vi "ShamStimSimple.vi"(0 "event in port":u16=5557, 5 "event in channel":u16=1 min=1 max=8, 7 "Digital sham stim channel":tag="PCI-DAQ/port0/line0") -> (4 "New event":bool, 6 "Time on (samp.)":i64, 8 "Crossing time":i64, 10 "Crossing level":sgl, 13 "Phase threshold":sgl(graph)=145.96965, 14 "Learning rate (for adaptive threshold)":dbl(graph)=0.005000000792214087)   [LabVIEW 2017]
uses:
  <vilib>/Platform/TimedLoop/XDataNode/timing_clust.ctl
  <vilib>/Platform/TimedLoop/XDataNode/nitl_modes.ctl
  <vilib>/Platform/TimedLoop/XDataNode/wakeup.ctl
  <vilib>/DAQmx/write.llb/DAQmx Write (Digital Bool 1Line 1Point).vi
  <vilib>/DAQmx/miscellaneous.llb/DAQmx Fill In Error Info.vi
  <vilib>/platform/TimedLoop/XDataNode/XDataNode.xnode
  <vilib>/addons/zeromq/zmq_socket.lvclass
  <vilib>/Platform/TimedLoop/XDataNode/XDNodeRunTimeDep.lvlib
panel:
  out "last run error":errorcluster
  in  "event out channel":u16=3
  in  "Output type":enum16{"DAQ Digital Out", "Network Event"}(ring)=enum."Network Event"
  in  "event out port":u16=5556
  in  "stop":bool
  in  "Run":bool
  # "*** Start OpenEphys acquisition before the VI. ***"
  # "*** In the audio settings in the OpenEphys GUI, reduce the buffer size to get a 10 ms buffer period.  If ASIO is installed and enabled in\nthe Open Ephys build, use ASIO with sample rate (in audio settings) = 192,000 Hz and buffer size = 192 (1 ms buffer period). ***"
  # "Settings only take effect\nnext time a run is started."
  # "If output type is \"Network Event\":"
  # "If output type is \"DAQ Digital Out\":"
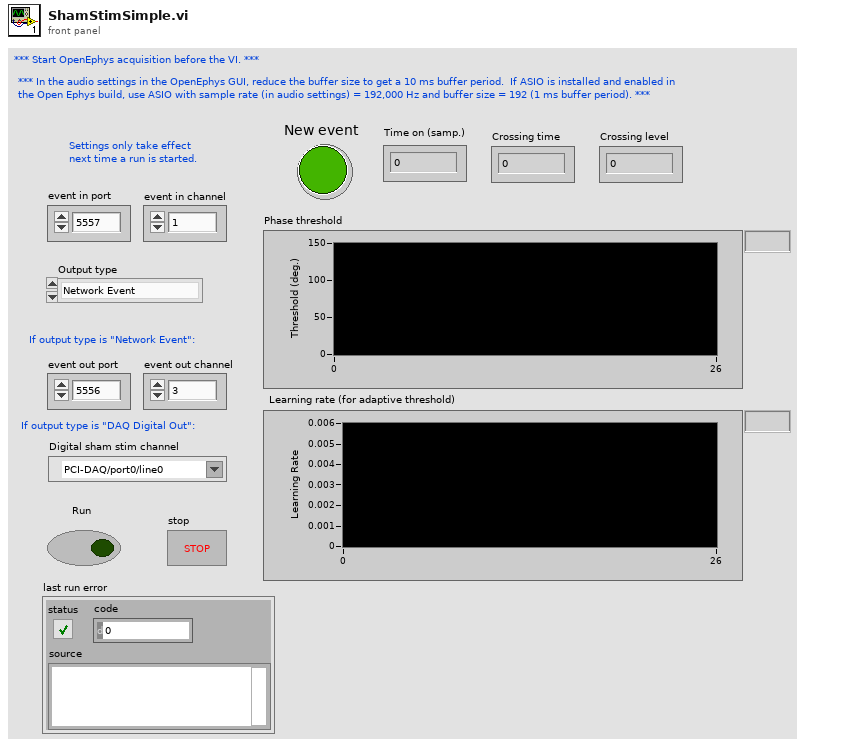
[diagram p1: front panel]
types:
  T1 = typedef "XDNodeRunTimeDep.lvlib/timing_clust.ctl" = cluster{"Expected End [f-1]":u64, "Actual End [f-1]":u64, "Finished Late? [f-1]":bool, "Expected End [i-1]":u64, "Actual End [i-1]":u64, "Finished Late? [i-1]":bool, "Expected Start [i]":u64, "Actual Start [i]":u64, "Expected Start [f]":u64, "Actual Start [f]":u64, "Source Name":string, "Structure Name":string, "Period":i64, "Deadline":i64, "Offset":i64, "Start":i64, "Priority":i32, "Timeout":i32, "Mode":T2, "Wakeup Reason":T3, "Error":errorcluster, "Source Type":string, "Secondary Source Type":string, "Global End Time":u64, "Global Start Time":u64, "Frame Duration":u64, "Iteration Duration":u64, "Assigned CPU":i32, "I/O Scan Engine Mode":u32}
  T2 = typedef "XDNodeRunTimeDep.lvlib/nitl_modes.ctl" = enum32{"No Change", "Process missed periods, maintain original phase", "Discard missed periods, maintain original phase", "Process missed periods, ignore original phase", "Discard missed periods, ignore original phase"}
  T3 = typedef "XDNodeRunTimeDep.lvlib/wakeup.ctl" = enum32{"Normal", "Aborted", "Asynchronous wakeup", "Timing source error", "Timed loop error", "Timeout"}
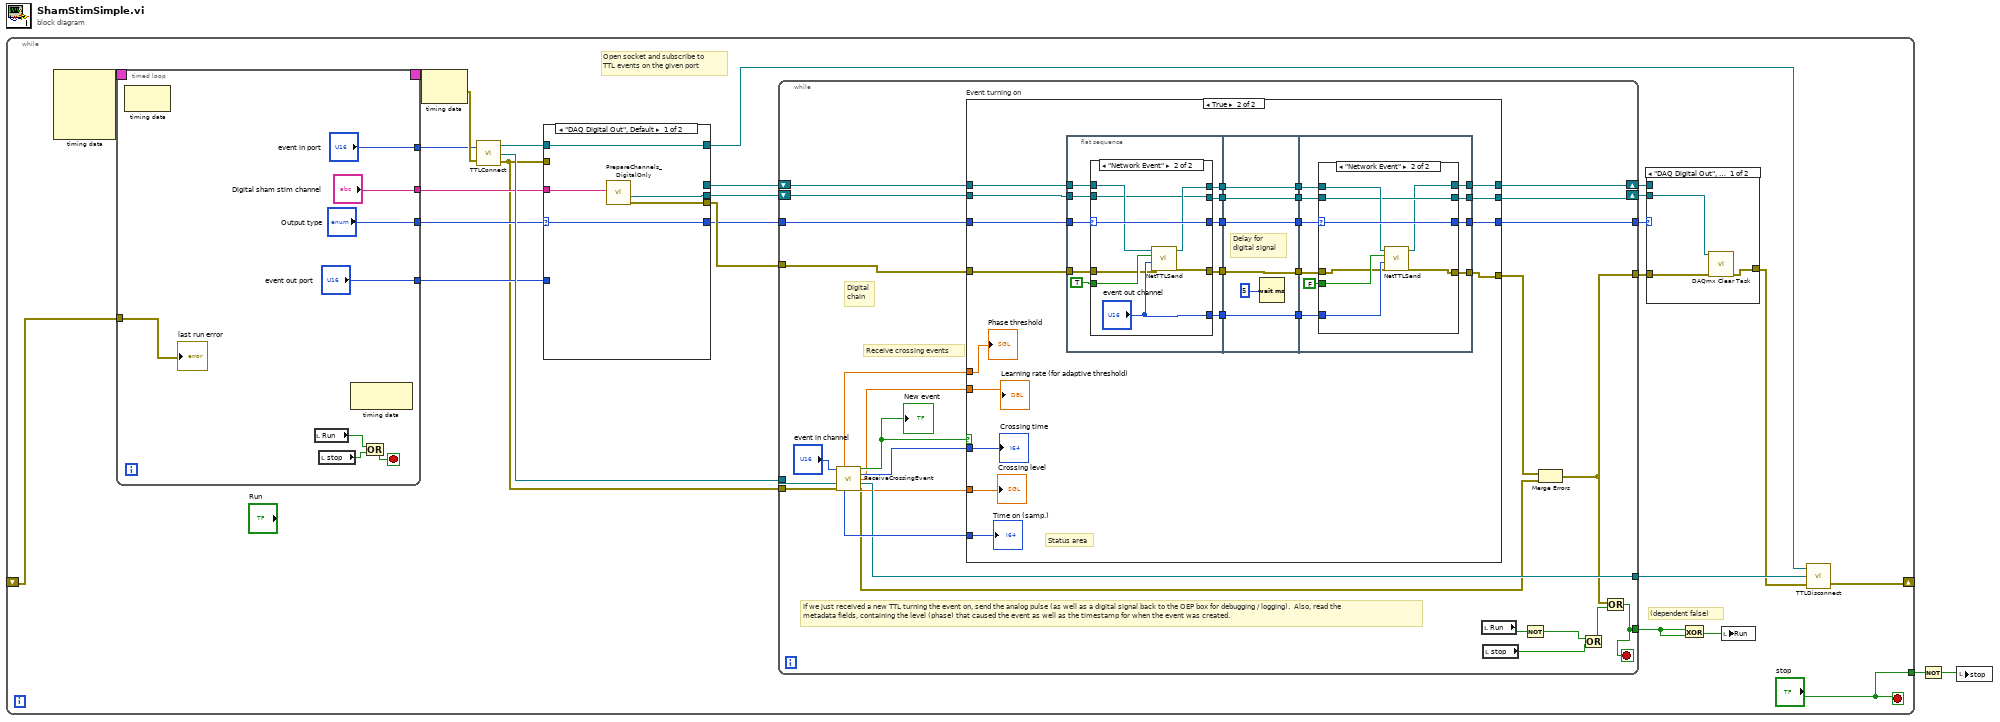
[diagram p0: block diagram]
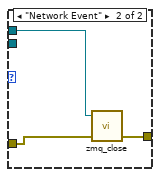
[diagram p2: hidden frame]
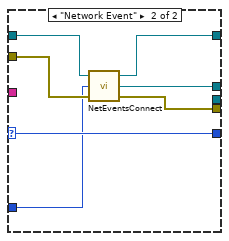
[diagram p3: hidden frame]
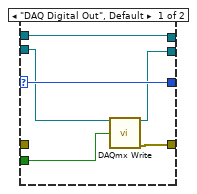
[diagram p5: hidden frame]
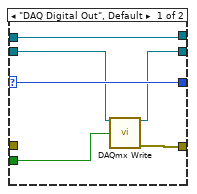
[diagram p6: hidden frame]
diagram:
  n1 = while {
    tunnel: ["stop"] -> w2
    shift-right: [w7] -> _
    shift-left: _ -> [w3]
    stop <- "stop" stop-if-true
    # "(dependent false)"
    # "Open socket and subscribe to\nTTL events on the given port"
    n2 = node-c288() -> (w28:T1)  [unwired: 4 in]
    n3 = timed-loop {
      timing: w28 -> [_]
      timing-out: [_] -> w27
      tunnel: ["event in port"] -> w23
      tunnel: ["event out port"] -> w17
      tunnel: ["Digital sham stim channel"] -> w22
      tunnel: ["Output type"] -> w20
      tunnel: w3 -> [w47]
      stop <- w52 stop-if-true
      n4 = node-c288() -> ()  [unwired: 1 in, 1 out]
      n5 = local read "Run"() -> (w53:bool)
      n6 = local read "stop"() -> (w54:bool)
      n7 = node-c288() -> ()  [unwired: 1 in, 1 out]
      n8 = Or(x=w53, y=w54) -> (x .or. y?=w52:bool)
      "last run error" <- w47
    }
    n9 = node-c288(w27) -> (w24:errorcluster)
    n10 = call "TTLConnect.vi"("port"=w23, "error in"=w24) -> ("context out"=w16:refnum<class "zmq_context.lvclass">, "socket out"=w25:refnum<class "zmq_socket.lvclass">, "error out"=w15:errorcluster)
    n11 = case shown="\"DAQ Digital Out\", Default" w20 {
      selector: w20 -> [w37 w46]
      tunnel: w22 -> [w39 _]
      tunnel: [w38 w43] -> w21
      tunnel: [w37 w46] -> w19
      tunnel: w17 -> [_ w41]
      tunnel: w15 -> [_ w42]
      tunnel: w16 -> [w36 w45]
      tunnel: [w36 w44] -> w14
      tunnel: [_ w40] -> w13
      tunnel: [w35 _] -> w12
      frame "DAQ Digital Out", Default {
        n12 = call "PrepareChannels_DigitalOnly.vi"("DO Physical channels"=w39) -> ("DO task out"=w35:refnum<k21>, "DO error out"=w38:errorcluster)  [unwired: 8 in]
      }
      frame "Network Event" {
        n13 = call "NetEventsConnect.vi"("error in"=w42, "port"=w41, "context in"=w45) -> ("error out"=w43:errorcluster, "socket out"=w40:refnum<class "zmq_socket.lvclass">, "context out"=w44:refnum<class "zmq_context.lvclass">)
      }
    }
    n14 = while {
      tunnel: [w81] -> w26
      tunnel: w25 -> [w74]
      tunnel: w21 -> [w70]
      tunnel: w19 -> [w69]
      tunnel: [w68] -> w18
      tunnel: w15 -> [w67]
      shift-right: [w63] -> w11
      shift-left: w13 -> [w66]
      shift-right: [w64] -> w10
      shift-left: w12 -> [w65]
      tunnel: [w61] -> w9
      tunnel: [w60] -> w5
      stop <- w60 stop-if-true
      # "Digital\nchain"
      # "If we just received a new TTL turning the event on, send the analog pulse (as well as a digital signal back to the OEP box for debugging / logging).  Also, read the metadata fields, containing the level (phase) that caused the event as well as the timestamp for when the event was created."
      # "Receive crossing events"
      n15 = call "ReceiveCrossingEvent.vi"("channel"="event in channel", "socket in"=w74, "error in"=w67) -> ("threshold"=w78:sgl, "new crossing"=w84:bool, "crossing time"=w83:i64, "learning rate"=w77:dbl, "socket out"=w81:refnum<class "zmq_socket.lvclass">, "event time"=w82:i64, "crossing level"=w80:sgl, "error out"=w75:errorcluster)  [unwired: 4 in, 1 out]
      "New event" <- w84
      n16 = case "Event turning on" shown="True" w84 {
        tunnel: w70 -> [w88 w111]
        tunnel: [w88 w105] -> w76
        tunnel: w83 -> [_ w109]
        tunnel: w82 -> [_ w110]
        tunnel: w80 -> [_ w108]
        tunnel: w78 -> [_ w107]
        tunnel: w77 -> [_ w106]
        tunnel: w69 -> [w87 w102]
        tunnel: [w87 w99] -> w68
        tunnel: w66 -> [w86 w96]
        tunnel: w65 -> [w85 w95]
        tunnel: [w85 w90] -> w64
        tunnel: [w86 w89] -> w63
        frame False {
        }
        frame True {
          # "Status area"
          n17 = flat-sequence {
            tunnel: [w120] -> w104
            tunnel: w111 -> [w121]
            tunnel: w102 -> [w119]
            tunnel: [w118] -> w100
            tunnel: [w116] -> w97
            tunnel: w96 -> [w115]
            tunnel: w95 -> [w113]
            tunnel: [w114] -> w93
            tunnel: [w112] -> w91
            tunnel: [w141] -> w103
            tunnel: w104 -> [w141]
            tunnel: [w139] -> w101
            tunnel: w100 -> [w139]
            tunnel: [w138] -> w98
            tunnel: w97 -> [w138]
            tunnel: [w137] -> w94
            tunnel: w93 -> [w137]
            tunnel: [w136] -> w92
            tunnel: w91 -> [w136]
            tunnel: w103 -> [w151]
            tunnel: [w150] -> w105
            tunnel: w101 -> [w148]
            tunnel: [w147] -> w99
            tunnel: w98 -> [w146]
            tunnel: w94 -> [w145]
            tunnel: w92 -> [w144]
            tunnel: [w143] -> w90
            tunnel: [w142] -> w89
            frame #0 {
              n18 = case shown="\"Network Event\"" w119 {
                selector: w119 -> [w126 w135]
                tunnel: w121 -> [_ w128]
                tunnel: [w127 w132] -> w120
                tunnel: [w126 w135] -> w118
                tunnel: TRUE ("data") -> [w125 w134]
                tunnel: [_ "event out channel"] -> w116
                tunnel: w115 -> [w124 w131]
                tunnel: [w124 w130] -> w114
                tunnel: [w122 w129] -> w112
                tunnel: w113 -> [w123 w129]
                frame "DAQ Digital Out", Default {
                  n19 = call-poly <vilib>:"DAQmx Write.vi"("task/channels in"=w123, "data"=w125) -> ("task out"=w122:refnum<k21>, "error out"=w127:errorcluster)  [unwired: 11 in, 1 out]
                }
                frame "Network Event" {
                  n20 = call "NetTTLSend.vi"("error in"=w128, "channel"="event out channel", "turn on?"=w134, "socket in"=w131) -> ("error out"=w132:errorcluster, "socket out"=w130:refnum<class "zmq_socket.lvclass">)  [unwired: 6 in]
                }
              }
            }
            frame #1 {
              # "Delay for \ndigital signal"
              n21 = Wait (ms)(milliseconds to wait=u32 5) -> ()  [unwired: 1 out]
            }
            frame #2 {
              n22 = case shown="\"Network Event\"" w148 {
                selector: w148 -> [w155 w163]
                tunnel: w151 -> [_ w158]
                tunnel: [w157 w164] -> w150
                tunnel: FALSE ("data") -> [w156 w162]
                tunnel: [w155 w163] -> w147
                tunnel: w146 -> [_ w165]
                tunnel: w145 -> [w154 w161]
                tunnel: [w152 w160] -> w143
                tunnel: w144 -> [w153 w160]
                tunnel: [w154 w159] -> w142
                frame "DAQ Digital Out", Default {
                  n23 = call-poly <vilib>:"DAQmx Write.vi"("task/channels in"=w153, "data"=w156) -> ("task out"=w152:refnum<k21>, "error out"=w157:errorcluster)  [unwired: 11 in, 1 out]
                }
                frame "Network Event" {
                  n24 = call "NetTTLSend.vi"("error in"=w158, "channel"=w165, "turn on?"=w162, "socket in"=w161) -> ("error out"=w164:errorcluster, "socket out"=w159:refnum<class "zmq_socket.lvclass">)  [unwired: 6 in]
                }
              }
            }
          }
          "Time on (samp.)" <- w110
          "Crossing time" <- w109
          "Crossing level" <- w108
          "Phase threshold" <- w107
          "Learning rate (for adaptive threshold)" <- w106
        }
      }
      n25 = local read "Run"() -> (w72:bool)
      n26 = local read "stop"() -> (w71:bool)
      n27 = Not(x=w72) -> (.not. x?=w73:bool)
      n28 = Merge Errors(w76, w75) -> (w61:errorcluster)
      n29 = Or(x=w73, y=w71) -> (x .or. y?=w62:bool)
      n30 = Or(x=w61, y=w62) -> (x .or. y?=w60:bool)
    }
    n31 = case shown="\"DAQ Digital Out\", Default" w18 {
      tunnel: w11 -> [_ w34]
      tunnel: w10 -> [w31 _]
      tunnel: [w30 w33] -> w8
      tunnel: w9 -> [w29 w32]
      frame "DAQ Digital Out", Default {
        n32 = call <vilib>:"DAQmx Clear Task.vi"("task in"=w31, "error in"=w29) -> ("error out"=w30:errorcluster)  [unwired: 13 in]
      }
      frame "Network Event" {
        n33 = call <vilib>:"zmq_close.vi"("error in"=w32, "socket"=w34) -> ("error out"=w33:errorcluster)  [unwired: 3 in]
      }
    }
    n34 = Exclusive Or(1:w5, 2:w5) -> (0:w4:bool)
    n35 = local write "Run"(w4) -> ()
    n36 = call "TTLDisconnect.vi"("error in"=w8, "socket in"=w26, "context in"=w14) -> ("error out"=w7:errorcluster)  [unwired: 1 in]
  }
  n37 = Not(x=w2) -> (.not. x?=w1:bool)
  n38 = local write "stop"(w1) -> ()
